vi "DestroySelfReference.vi"(8 "error in (no error)":errorcluster, 11 "SMO":refnum<class "SMO.lvclass">) -> (0 "error out":errorcluster, 3 "SMO out":refnum<class "SMO.lvclass">)   [LabVIEW 2013, in "SMO.lvclass"]
uses:
  SMO.lvclass
  SMO.lvclass/SMO.ctl
panel:
  # "For instructions on how to use the JKI State Machine Objects, examples and video tutorials, visit:\nhttp://jki.net/state-machine-objects/\n\nJKI State Machine Objects™\nhttp://jki.net/state-machine-objects/\nCopyright (C) 2005-2015, JKI <info@jki.net>\nALL RIGHTS RESERVED"
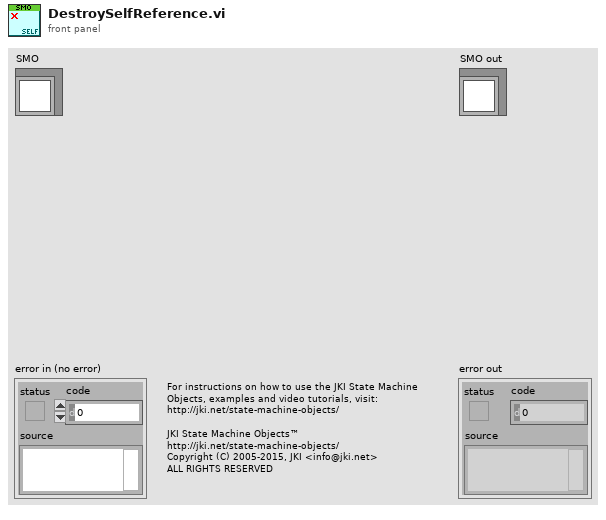
[diagram p1: front panel]
types:
  T1 = typedef "SMO.lvclass/PrivateData--Ref.ctl" = refnum<data-value>
  T2 = typedef "SMO.lvclass/PrivateData--Cluster.ctl" = cluster{"Parent Call":T3, "Registered Processes":T4[], "Sync Notifier":refnum<notifier>, "Process Error Notifier":refnum<notifier>, "Protected Events":T5, "Public Events":T6, "SMO State":T7, "[Dependencies]":T8[], "[Attributes]":refnum<class "Attribute.lvclass">[], "Launcher Close":refnum<notifier>, "Caller Watchdog":refnum<queue>}
  T3 = typedef "SMO.lvclass/Parent Call--Enum.ctl" = enum16{"Allows parent to run", "Does not request parent to run"}
  T4 = typedef "SMO.lvclass/RegisteredProcessData--Cluster.ctl" = cluster{"Name":string, "Static VI Ref":refnum<vi>, "Running":bool, "NotifierRef":u32}
  T5 = typedef "SMO.lvclass/Protected Events.ctl" = cluster{"StopProcesses":refnum<user-event>, "AbortProcesses":refnum<user-event>, "Config Changed":refnum<user-event>, "Dependency":refnum<user-event>}
  T6 = typedef "SMO.lvclass/Public Events.ctl" = cluster{"Error":refnum<user-event>, "State":refnum<user-event>}
  T7 = typedef "SMO.lvclass/SMOState --Enum.ctl" = enum16{"unknown", "Created", "Started", "Stopped"}
  T8 = typedef "SMO.lvclass/SMO Dependency--Cluster.ctl" = cluster{"Dependency":refnum<class "SMO.lvclass">, "Level":string}
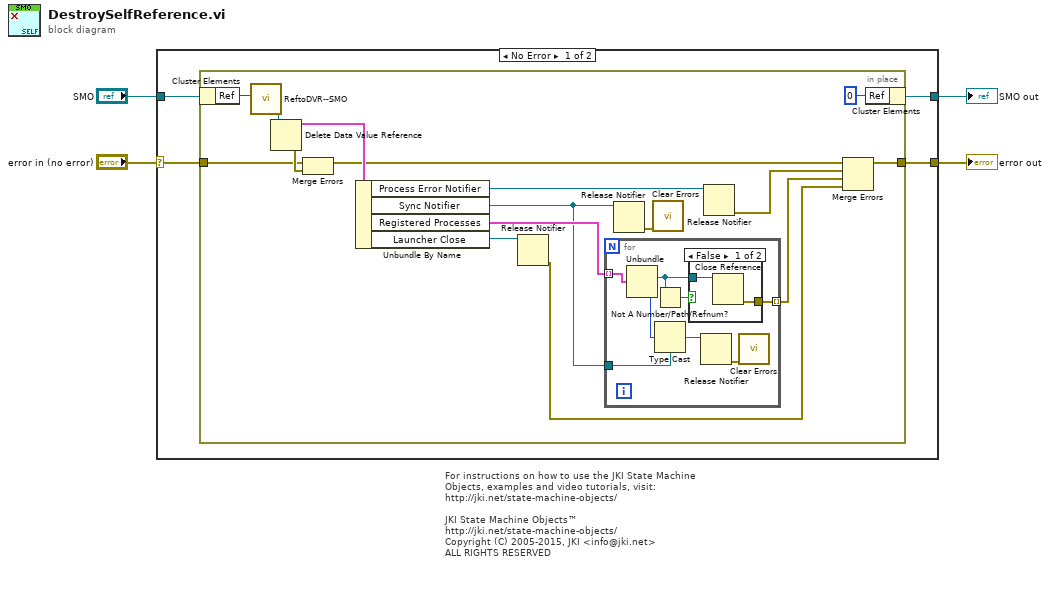
[diagram p0: block diagram]
diagram:
  # "For instructions on how to use the JKI State Machine Objects, examples and video tutorials, visit:\nhttp://jki.net/state-machine-objects/\n\nJKI State Machine Objects™\nhttp://jki.net/state-machine-objects/\nCopyright (C) 2005-2015, JKI <info@jki.net>\nALL RIGHTS RESERVED"
  n1 = case shown="No Error" "error in (no error)" {
    selector: "error in (no error)" -> [w8 w36]
    tunnel: [w7 w36] -> w3
    tunnel: [w5 w35] -> w1
    tunnel: "SMO" -> [w6 w35]
    frame No Error {
      n2 = in-place {
        in-place-border: w8 -> [w17]
        in-place-border: [w24] -> w7
        n3 = in-place-cluster #1(w6) -> ("Ref"=w14:u32)
        n4 = call "ReftoDVR--SMO.vi"("Ref"=w14) -> ("Ref"=w13:T1)  [unwired: 10 in]
        n5 = Delete Data Value Reference(data value reference=w13) -> (data value=w21:T2, error out=w18:errorcluster)  [unwired: 1 in]
        n6 = Merge Errors(w17, w18) -> (w16:errorcluster)
        n7 = Unbundle By Name(w21) -> ("Process Error Notifier"=w22:refnum<notifier>, "Sync Notifier"=w11:refnum<notifier>, "Registered Processes"=w23:T4[], "Launcher Close"=w10:refnum<notifier>)
        n8 = Release Notifier(notifier=w10) -> (error out=w9:errorcluster)  [unwired: 2 in, 2 out]
        n9 = for {
          tunnel: w23 -> [w31] mode=indexing
          tunnel: [w29] -> w19 mode=indexing
          tunnel: w11 -> [w27]
          n10 = Unbundle(w31) -> ("Static VI Ref"=w30:refnum<vi>, "NotifierRef"=w28:u32)  [unwired: 2 out]
          n11 = Not A Number/Path/Refnum?(number/path/refnum=w30) -> (NaN/Path/Refnum?=w32:bool)
          n12 = Type Cast(type=w27, x=w28) -> (*(type *) &x=w26:refnum<notifier>)
          n13 = case shown="False" w32 {
            tunnel: w30 -> [w34 _]
            tunnel: [w33 _] -> w29
            frame False {
              n14 = Close Reference(reference=w34) -> (error out=w33:errorcluster)  [unwired: 1 in]
            }
            frame True {
            }
          }
          n15 = Release Notifier(notifier=w26) -> (error out=w25:errorcluster)  [unwired: 2 in, 2 out]
          n16 = call <vilib>:"Clear Errors.vi"("error in (no error)"=w25) -> ()  [unwired: 6 in, 1 out]
        }
        n17 = Release Notifier(notifier=w11) -> (error out=w12:errorcluster)  [unwired: 2 in, 2 out]
        n18 = call <vilib>:"Clear Errors.vi"("error in (no error)"=w12) -> ()  [unwired: 6 in, 1 out]
        n19 = Release Notifier(notifier=w22) -> (error out=w20:errorcluster)  [unwired: 2 in, 2 out]
        n20 = Merge Errors(w16, w20, w19, w9) -> (w24:errorcluster)
        n21 = in-place-cluster #1("Ref"=u32 0) -> (w5:refnum<class "SMO.lvclass">)
      }
    }
    frame Error {
    }
  }
  "error out" <- w3
  "SMO out" <- w1
